vi "Unflatten Value.vi"(8 "Error In":errorcluster, 10 "Value":string, 11 "StringArray In":refnum<class "1D String.lvclass">) -> (0 "Error Out":errorcluster, 3 "StringArray Out":refnum<class "1D String.lvclass">)   [LabVIEW 2020, in "NI_VIAnCFGDataStructure.lvlib" / "1D String.lvclass"]
uses:
  <vilib>/addons/analyzer/VIAnCFGDataStructure/Data Types/String Array/1D String.lvclass
  <vilib>/addons/analyzer/VIAnCFGDataStructure/Data Types/String Array/1D String.lvclass/1D String.ctl
  <vilib>/addons/analyzer/VIAnCFGDataStructure/Tree Manager/API/Generate Hash.vi
  <vilib>/regexp/Match Regular Expression.xnode
  <vilib>/addons/analyzer/VIAnCFGDataStructure/Tree Manager/Tree.lvclass
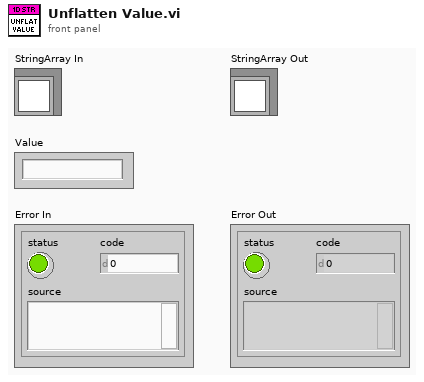
[diagram p1: front panel]
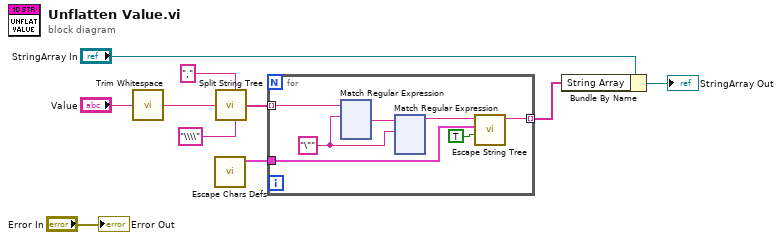
[diagram p0: block diagram]
diagram:
  n1 = call <vilib>:"Trim Whitespace.vi"("string"="Value") -> ("trimmed string"=w1:string)  [unwired: 1 in]
  n2 = call <vilib>:"Escape Chars Defs.vi"() -> ("Escapes"=w7:cluster{"String":string, "Escape":string}[])  [unwired: 11 in]
  n3 = call <vilib>:"Split String Tree.vi"("Ignore Pattern"="\\\\", "Split Pattern"=",", "Input String"=w1) -> ("Split String"=w5:string[])  [unwired: 4 in]
  n4 = for {
    tunnel: w5 -> [w14] mode=indexing
    tunnel: [w15] -> w4 mode=indexing
    tunnel: w7 -> [w17]
    w12 = "\"" ("regular expression")
    n5 = xnode "Match Regular Expression"("input string"=w14, "regular expression"=w12) -> ("after match"=w13:string)  [unwired: 4 in, 4 out]
    n6 = xnode "Match Regular Expression"("input string"=w13, "regular expression"=w12) -> ("before match"=w11:string)  [unwired: 4 in, 4 out]
    n7 = call <vilib>:"Escape String Tree.vi"("Reverse? (False)"=TRUE ("Remove Escapes? (False)"), "Escapes"=w17, "String In"=w11) -> ("String Out"=w15:string)  [unwired: 8 in]
  }
  n8 = Bundle By Name(cluster="StringArray In", "String Array"=w4) -> (→"StringArray Out":refnum<class "1D String.lvclass">)
  "Error Out" <- "Error In"
